vi "rqp_Disconnect Server.vi"(4 "Show in Debugger?":bool=TRUE, 6 "Message Priority":T1=enum."Normal", 7 "Caller in":refnum<class "Worker.lvclass">, 8 "error in":errorcluster, 11 "TCP Client in":refnum<class "TCP Client.lvclass">) -> (0 "error out":errorcluster, 3 "dup TCP Client out":refnum<class "TCP Client.lvclass">, 5 "dup Caller out":refnum<class "Worker.lvclass">)   [LabVIEW 2017, in "_TCP Client.lvlib" / "TCP Client.lvclass"]
doc: "This VI sends a <b>Public API Request</b> message to an MHL case of the Worker that owns this VI.\n---\nDisconnects the TCP Client connection to the TCP Server."
uses:
  TCP Client.lvclass
  C:/SC/Source Code/VIPM/LabVIEW 20xx/vi.lib/addons/_Workers/Library/Classes/Worker/Worker.lvclass
  <vilib>/addons/_Workers/Library/Classes/Worker/Worker.lvclass
  <vilib>/addons/_Workers/Library/Classes/Message/Priority.ctl
  <vilib>/addons/_Workers/Library/Case Label.ctl
  rqp_Disconnect Server.ctl
  <vilib>/addons/_Workers/Library/Classes/Message Queue/Message Queue.lvclass
  <vilib>/addons/_Workers/Library/Workers.lvlib
  <vilib>/addons/_Workers/Library/Classes/Message/Message.lvclass
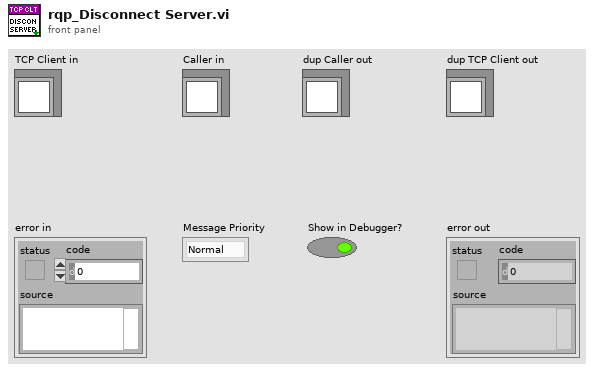
[diagram p1: front panel]
types:
  T1 = typedef "Workers.lvlib/Message.lvclass/Priority.ctl" = enum16{"Low", "Normal", "High"}
  T2 = typedef "_TCP Client.lvlib/TCP Client.lvclass/rqp_Disconnect Server.ctl" = cluster{"String":string}
  T3 = typedef "Workers.lvlib/Case Label.ctl" = string
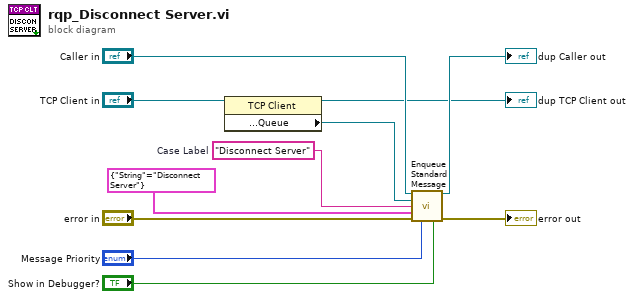
[diagram p0: block diagram]
diagram:
  w1 = T3 "Disconnect Server"  # Case Label
  n1 = property class="TCP Client"(reference="TCP Client in") -> (reference out=→"dup TCP Client out":refnum<class "TCP Client.lvclass">, "Accessors:Read:Public API:Queue"=w2:refnum<class "Message Queue.lvclass">)  [unwired: 1 in, 1 out]
  n2 = call-dynamic "Enqueue Standard Message.vi"("Worker"="Caller in", "Message Queue"=w2, "Case Label"=w1, "Data"=T2 {"String"="Disconnect Server"} ("Data in"), "error in (no error)"="error in", "Priority (Normal)"="Message Priority", "Send Message to Debugger? (T)"="Show in Debugger?") -> ("dup Worker out"=→"dup Caller out":refnum<class "Worker.lvclass">, "error out"=→"error out":errorcluster)  [unwired: 7 in]
